vi "stringtoint32.vi"(11 "input_string":string) -> (3 "output_int":u32 format="%x")   [LabVIEW 2014]
panel:
  out "number 4":u32 format="%x"
  out "number 3":u32 format="%x"
  out "number 2":u32 format="%x"
  out "number":u32 format="%x"
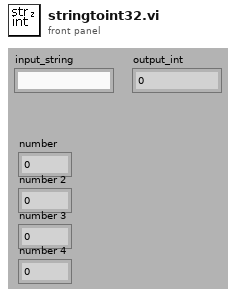
[diagram p1: front panel]
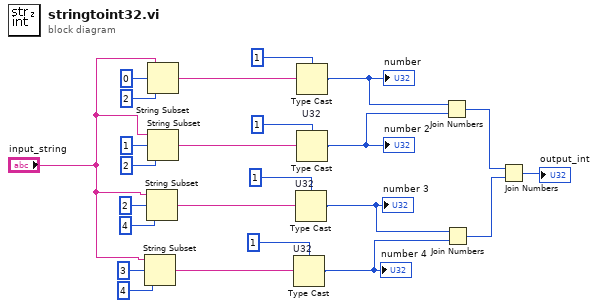
[diagram p0: block diagram]
diagram:
  n1 = String Subset(string="input_string", offset (0)=3, length (rest)=4 ("length (rest)")) -> (substring=w11:string)
  n2 = String Subset(string="input_string", offset (0)=2, length (rest)=4 ("length (rest)")) -> (substring=w12:string)
  n3 = String Subset(string="input_string", offset (0)=0, length (rest)=2 ("length (rest)")) -> (substring=w21:string)
  n4 = String Subset(string="input_string", offset (0)=1, length (rest)=2 ("length (rest)")) -> (substring=w20:string)
  n5 = Type Cast "U32"(type=u8 1 ("Numeric"), x=w11) -> (*(type *) &x=w4:u8)
  "number 4" <- w4
  n6 = Type Cast "U32"(type=u8 1 ("Numeric"), x=w12) -> (*(type *) &x=w5:u8)
  "number 3" <- w5
  n7 = Type Cast(type=u8 1 ("Numeric"), x=w21) -> (*(type *) &x=w16:u8)
  "number" <- w16
  n8 = Type Cast "U32"(type=u8 1 ("Numeric"), x=w20) -> (*(type *) &x=w15:u8)
  "number 2" <- w15
  n9 = Join Numbers(hi=w16, lo=w15) -> ((hi.lo)=w6:u16)
  n10 = Join Numbers(hi=w5, lo=w4) -> ((hi.lo)=w3:u16)
  n11 = Join Numbers(hi=w6, lo=w3) -> ((hi.lo)=→"output_int":u32)
